vi "Example Graph.vi"() -> ()   [LabVIEW 2013]
uses:
  C:/tf/play/labview/Tinkerforge.dll
  Tinkerforge.dll
panel:
  in  "stop":bool
  out "graph":i16[](graph)
  in  "uid":string="8e7"
  in  "port":i32=4223
  in  "host":string="localhost"
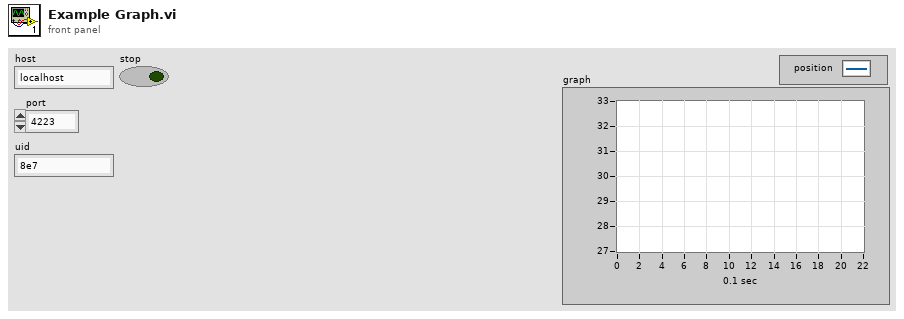
[diagram p1: front panel]
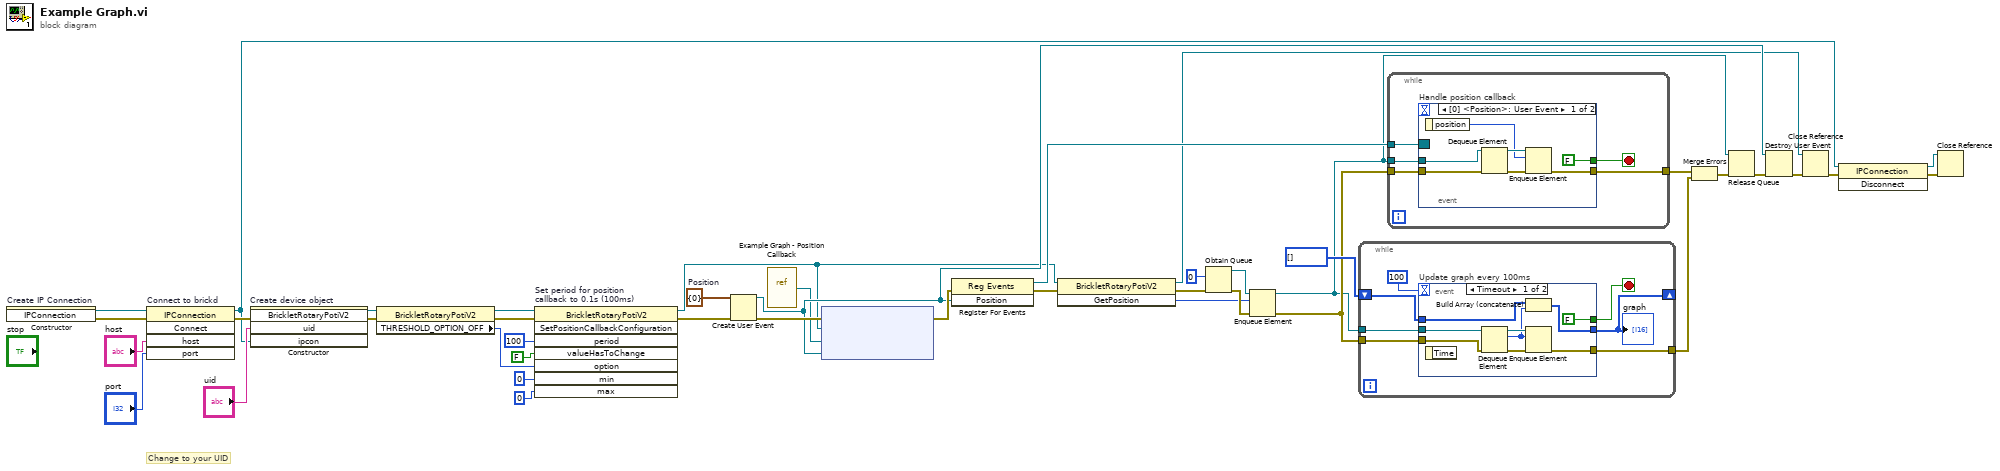
[diagram p0: block diagram]
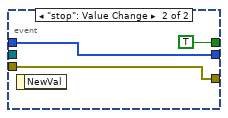
[diagram p2: hidden frame]
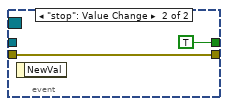
[diagram p3: hidden frame]
diagram:
  w28 = cluster{"position":i16} {"position"=0}  # Position
  # "Change to your UID"
  n1 = constructor on="Create IP Connection" class="IPConnection"() -> (reference out=w42:refnum<k24>, error out=w15:errorcluster)  [unwired: 3 in, 1 out]
  n2 = invoke on="Connect to brickd" class="IPConnection" method="Connect"(reference=w42, error in=w15, "host"="host", "port"="port") -> (reference out=w35:refnum<k24>, error out=w38:errorcluster)  [unwired: 1 in, 3 out]
  n3 = constructor on="Create device object" class="BrickletRotaryPotiV2"(error in=w38, "uid"="uid", "ipcon"=w35) -> (reference out=w6:refnum<k24>, error out=w3:errorcluster)  [unwired: 2 in, 3 out]
  n4 = property class="BrickletRotaryPotiV2"(reference=w6, error in=w3) -> (reference out=w5:refnum<k24>, error out=w2:errorcluster, "THRESHOLD_OPTION_OFF"=w4:u16)
  n5 = invoke on="Set period for position\ncallback to 0.1s (100ms)" class="BrickletRotaryPotiV2" method="SetPositionCallbackConfiguration"(reference=w5, error in=w2, "period"=i64 100, "valueHasToChange"=FALSE, "option"=w4, "min"=i16 0, "max"=i16 0) -> (reference out=w12:refnum<k24>, error out=w27:errorcluster)  [unwired: 1 in, 6 out]
  n6 = Create User Event(user event datatype=w28, error in=w27) -> (user event=w30:refnum<user-event>, error out=w33:errorcluster)
  n7 = vi-ref "Example Graph - Position Callback.vi"() -> ("vi reference"=w1:refnum<vi>)
  n8 = node ("Register Event Callback")(w33, w12, w1, w30) -> (w32:errorcluster)  [unwired: 1 in, 1 out]
  n9 = register-events(error in=w32, w30) -> (reference out=w31:refnum<event-registration>, error out=w14:errorcluster)  [unwired: 1 in]
  n10 = invoke class="BrickletRotaryPotiV2" method="GetPosition"(reference=w12, error in=w14) -> (reference out=w11:refnum<k24>, error out=w13:errorcluster, "GetPosition"=w10:i16)  [unwired: 1 in]
  n11 = Obtain Queue(element data type=i16 0, error in (no error)=w13) -> (queue out=w19:refnum<queue>, error out=w21:errorcluster)  [unwired: 3 in, 1 out]
  n12 = Enqueue Element(queue=w19, element=w10, error in (no error)=w21) -> (queue out=w16:refnum<queue>, error out=w20:errorcluster)  [unwired: 1 in, 1 out]
  n13 = while {
    tunnel: [w45] -> w25
    tunnel: w20 -> [w46]
    shift-right: [w47] -> _
    shift-left: i16[] [] -> [w48]
    tunnel: w16 -> [w44]
    stop <- w43 stop-if-true
    n14 = event "Update graph every 100ms" shown="[0] Timeout" {
      selector: _ -> [_ _]
      dyn-events: _ -> [_ _]
      timeout: 100 -> [_ _]
      tunnel: [w58 w60] -> w47
      tunnel: w48 -> [w51 w60]
      tunnel: w46 -> [w57 w59]
      tunnel: [w54 w59] -> w45
      tunnel: w44 -> [w56 _]
      tunnel: [FALSE TRUE] -> w43
      event Timeout {
        n15 = event-data() -> ()  [unwired: 1 in, 1 out]
        n16 = Dequeue Element(queue=w56, error in (no error)=w57) -> (queue out=w53:refnum<queue>, element=w52:i16, error out=w55:errorcluster)  [unwired: 1 in, 1 out]
        n17 = Build Array (concatenate)(w51, w52) -> (w58:i16[])
        n18 = Enqueue Element(queue=w53, element=w52, error in (no error)=w55) -> (error out=w54:errorcluster)  [unwired: 1 in, 2 out]
      }
      event "stop": Value Change {
        n19 = event-data() -> ()  [unwired: 1 in, 1 out]
      }
    }
    "graph" <- w47
  }
  n20 = while {
    tunnel: w31 -> [w66]
    tunnel: [w64] -> w24
    tunnel: w20 -> [w65]
    tunnel: w16 -> [w63]
    stop <- w62 stop-if-true
    n21 = event "Handle position callback" shown="[0] <Position>: User Event" {
      selector: w66 -> [_ _]
      dyn-events: _ -> [_ _]
      timeout: _ -> [_ _]
      tunnel: w65 -> [w73 w74]
      tunnel: [w71 w74] -> w64
      tunnel: w63 -> [w70 _]
      tunnel: [FALSE TRUE] -> w62
      event User Event {
        n22 = event-data() -> ("position"=w67:i16)  [unwired: 1 in]
        n23 = Dequeue Element(queue=w70, error in (no error)=w73) -> (queue out=w69:refnum<queue>, error out=w72:errorcluster)  [unwired: 1 in, 2 out]
        n24 = Enqueue Element(queue=w69, element=w67, error in (no error)=w72) -> (error out=w71:errorcluster)  [unwired: 1 in, 2 out]
      }
      event "stop": Value Change {
        n25 = event-data() -> ()  [unwired: 1 in, 1 out]
      }
    }
  }
  n26 = Merge Errors(w24, w25) -> (w18:errorcluster)
  n27 = Release Queue(queue=w16, error in (no error)=w18) -> (error out=w17:errorcluster)  [unwired: 1 in, 2 out]
  n28 = Destroy User Event(user event=w30, error in=w17) -> (error out=w29:errorcluster)
  n29 = Close Reference(reference=w11, error in (no error)=w29) -> (error out=w37:errorcluster)
  n30 = invoke class="IPConnection" method="Disconnect"(reference=w35, error in=w37) -> (reference out=w34:refnum<k24>, error out=w36:errorcluster)  [unwired: 1 in, 1 out]
  n31 = Close Reference(reference=w34, error in (no error)=w36) -> ()  [unwired: 1 out]
